vi "Initialize Instrument.vi"(8 "error in (no error)":errorcluster, 10 "Reset":bool, 11 "SigGen-SMBV in":refnum<class "VSG-SMBV.lvclass">) -> (0 "error out":errorcluster, 3 "SigGen-SMBV out":refnum<class "VSG-SMBV.lvclass">)   [LabVIEW 2020, in "VSG-SMBV.lvclass"]
uses:
  VSG-SMBV.lvclass
  C:/Sandbox/RF Bench/Source Code/WiSpry Test Framework/Instruments/Instrument.lvclass
  Instrument.lvclass/Instrument.ctl
  Instrument.lvclass
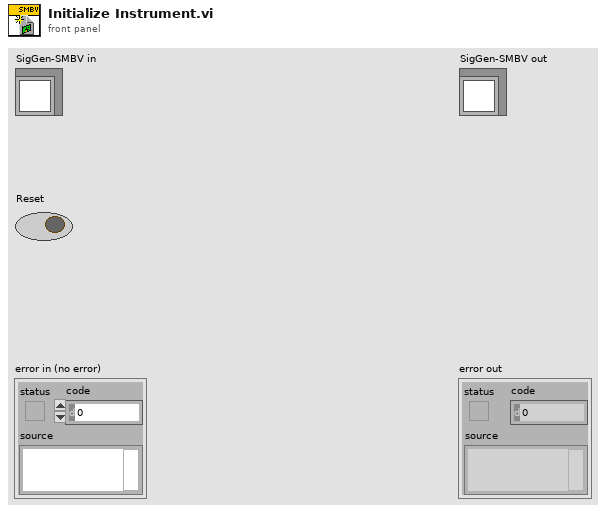
[diagram p1: front panel]
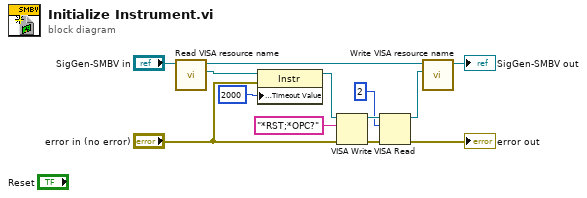
[diagram p0: block diagram]
diagram:
  n1 = call "Read VISA resource name.vi"("Instrument in"="SigGen-SMBV in") -> ("VISA resource name"=w9:refnum<visa-resource-name>, "Instrument out"=w7:refnum<class "VSG-SMBV.lvclass">)  [unwired: 9 in]
  n2 = property class="Instr"(reference=w9, error in="error in (no error)", "General Settings:Timeout Value"=u32 2000) -> (reference out=w8:refnum<visa-resource-name>)  [unwired: 1 out]
  n3 = VISA Write(VISA resource name=w8, write buffer="*RST;*OPC?", error in (no error)="error in (no error)") -> (VISA resource name out=w4:refnum<visa-resource-name>, error out=w5:errorcluster)  [unwired: 1 out]
  n4 = VISA Read(VISA resource name=w4, byte count=u32 2, error in (no error)=w5) -> (VISA resource name out=w1:refnum<visa-resource-name>, error out=→"error out":errorcluster)  [unwired: 2 out]
  n5 = call "Write VISA resource name.vi"("VISA resource name"=w1, "Instrument in"=w7) -> ("Instrument out"=→"SigGen-SMBV out":refnum<class "VSG-SMBV.lvclass">)  [unwired: 9 in]
